vi "实验4.vi"() -> ()   [LabVIEW 2014]
uses:
  <vilib>/Analysis/NI_AALPro.lvlib
panel:
  out "i":dbl
  out "瞬时标准电阻电压":dbl
  out "瞬时总电压":dbl
  in  "开关":bool
  out "数据":dbl[][](array[numeric])
  out "待测电阻值":dbl
  in  "时间间隔":dbl[unit]
  in  "标准电阻":dbl
  in  "测量数据点数":dbl
  in  "输出电压步长":dbl[unit]
  out "XY Graph":cluster{"Y":dbl[], "Y":dbl[]}[](graph) caption="电阻的伏安曲线图"
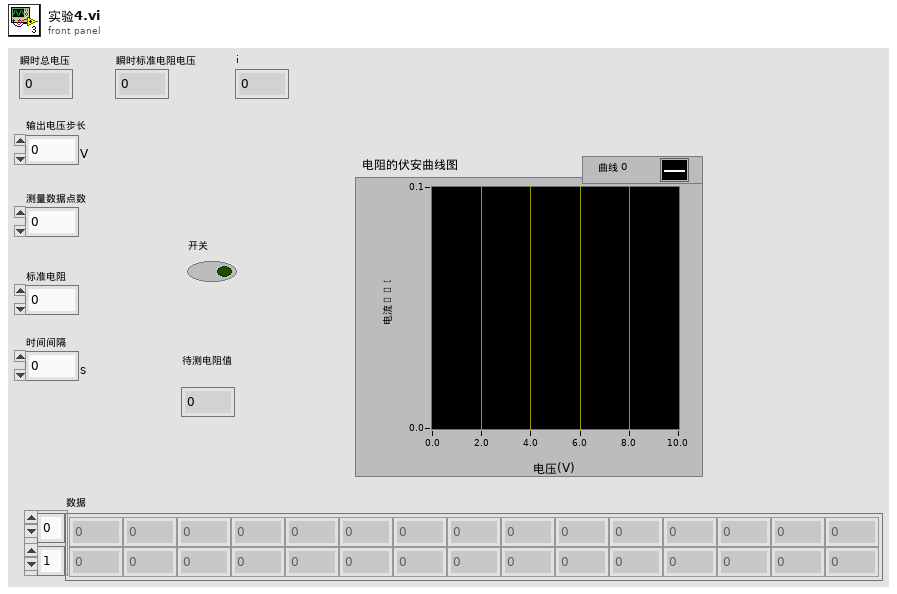
[diagram p1: front panel]
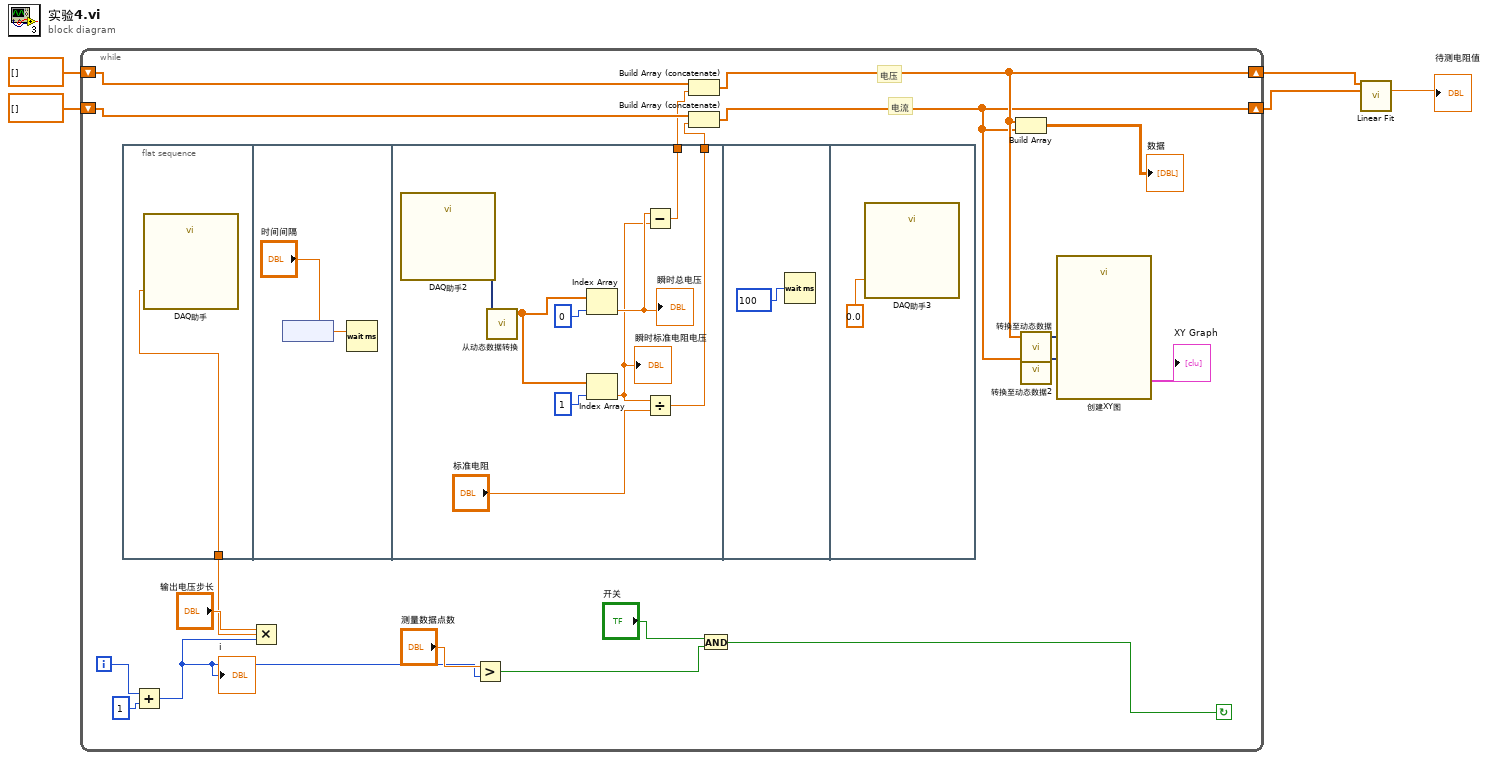
[diagram p0: block diagram]
diagram:
  n1 = while {
    shift-right: [w11] -> w2
    shift-left: dbl[] [] -> [w17]
    shift-right: [w13] -> w3
    shift-left: dbl[] [] -> [w18]
    i -> [w8]
    stop <- w14 continue-if-true
    # "电流"
    # "电压"
    n2 = flat-sequence {
      tunnel: w22 -> [w25]
      tunnel: [w31] -> w16
      tunnel: [w30] -> w15
      frame #0 {
        n3 = call "DAQ助手"("data"=w25) -> ()  [unwired: 17 in, 2 out]
      }
      frame #1 {
        n4 = node("时间间隔") -> (w26:dbl)
        n5 = Wait (ms)(milliseconds to wait=w26) -> ()  [unwired: 1 out]
      }
      frame #2 {
        n6 = call "DAQ助手2"() -> ("data"=w36:dynamicdata)  [unwired: 17 in, 2 out]
        n7 = call "从动态数据转换"("Dynamic Data Type"=w36) -> ("Array"=w35:dbl[])  [unwired: 3 in]
        n8 = Index Array(array=w35, index=0) -> (element=w29:dbl)
        "瞬时总电压" <- w29
        n9 = Index Array(array=w35, index=1) -> (element=w28:dbl)
        "瞬时标准电阻电压" <- w28
        n10 = Subtract(x=w29, y=w28) -> (x-y=w31:dbl)
        n11 = Divide(x=w28, y="标准电阻") -> (x/y=w30:dbl)
      }
      frame #3 {
        n12 = Wait (ms)(milliseconds to wait=100) -> ()  [unwired: 1 out]
      }
      frame #4 {
        n13 = call "DAQ助手3"("data"=0.0) -> ()  [unwired: 17 in, 2 out]
      }
    }
    n14 = Add(x=w8, y=1) -> (x+y=w6:i32)
    "i" <- w6
    n15 = Multiply(x="输出电压步长", y=w6) -> (x*y=w22:dbl[unit])
    n16 = Greater?(x="测量数据点数", y=w6) -> (0:w19:bool)
    n17 = Build Array (concatenate)(w18, w16) -> (w13:dbl[])
    n18 = Build Array (concatenate)(w17, w15) -> (w11:dbl[])
    n19 = And(x="开关", y=w19) -> (x .and. y?=w14:bool)
    n20 = Build Array(w13, w11) -> (→"数据":dbl[][])
    n21 = call "转换至动态数据"("Array"=w13) -> ("Dynamic Data Type"=w12:dynamicdata)  [unwired: 3 in]
    n22 = call "转换至动态数据2"("Array"=w11) -> ("Dynamic Data Type"=w10:dynamicdata)  [unwired: 3 in]
    n23 = call "创建XY图"("Y Input"=w10, "X Input"=w12) -> ("XY Graph"=→"XY Graph":cluster{"X":dbl[], "Y":dbl[]}[])  [unwired: 8 in, 1 out]
  }
  n24 = call <vilib>:"Linear Fit.vi"("Y"=w3, "X"=w2) -> ("slope"=→"待测电阻值":dbl)  [unwired: 9 in, 4 out]
